vi "Unit conversion.vi"(8 "error in (no error)":errorcluster, 9 "To(T) or From(F) Encoder":bool, 10 "value in":dbl, 11 "Motor in":refnum<class "Motor.lvclass">) -> (0 "error out":errorcluster, 2 "value out":dbl, 3 "Motor out":refnum<class "Motor.lvclass">)   [LabVIEW 2018, in "Motor.lvclass"]
uses:
  Motor.lvclass
  Motor.lvclass/Motor.ctl
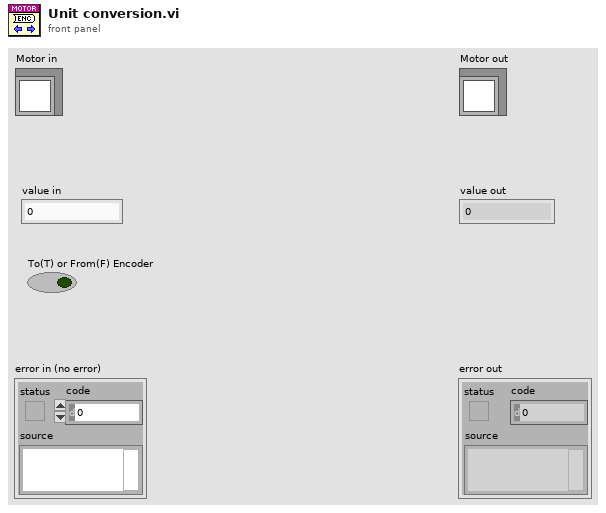
[diagram p1: front panel]
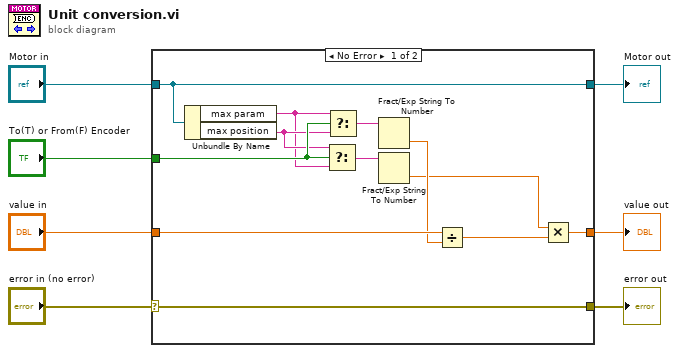
[diagram p0: block diagram]
diagram:
  n1 = case shown="No Error" "error in (no error)" {
    selector: "error in (no error)" -> [w19 w20]
    tunnel: [w19 w20] -> w6
    tunnel: [w18 w21] -> w4
    tunnel: "Motor in" -> [w18 w21]
    tunnel: "To(T) or From(F) Encoder" -> [w12 _]
    tunnel: "value in" -> [w17 _]
    tunnel: [w16 _] -> w1
    frame No Error {
      n2 = Unbundle By Name(w18) -> ("max param"=w8:string, "max position"=w9:string)
      n3 = Select(t=w9, s=w12, f=w8) -> (s? t:f=w10:string)
      n4 = Select(t=w8, s=w12, f=w9) -> (s? t:f=w11:string)
      n5 = Fract/Exp String To Number(string=w11) -> (number=w14:dbl)  [unwired: 3 in, 1 out]
      n6 = Fract/Exp String To Number(string=w10) -> (number=w13:dbl)  [unwired: 3 in, 1 out]
      n7 = Divide(x=w17, y=w14) -> (x/y=w15:dbl)
      n8 = Multiply(x=w13, y=w15) -> (x*y=w16:dbl)
    }
    frame Error {
    }
  }
  "error out" <- w6
  "Motor out" <- w4
  "value out" <- w1
